vi "pp_loadStimList.vi"(4 "error in (no error)":errorcluster) -> (0 "error out":errorcluster, 2 "Path":path, 3 "Stimulus List":dbl[][](array[numeric]))   [LabVIEW 2013]
uses:
  <vilib>/Utility/xml.llb/Read From XML File(array).vi
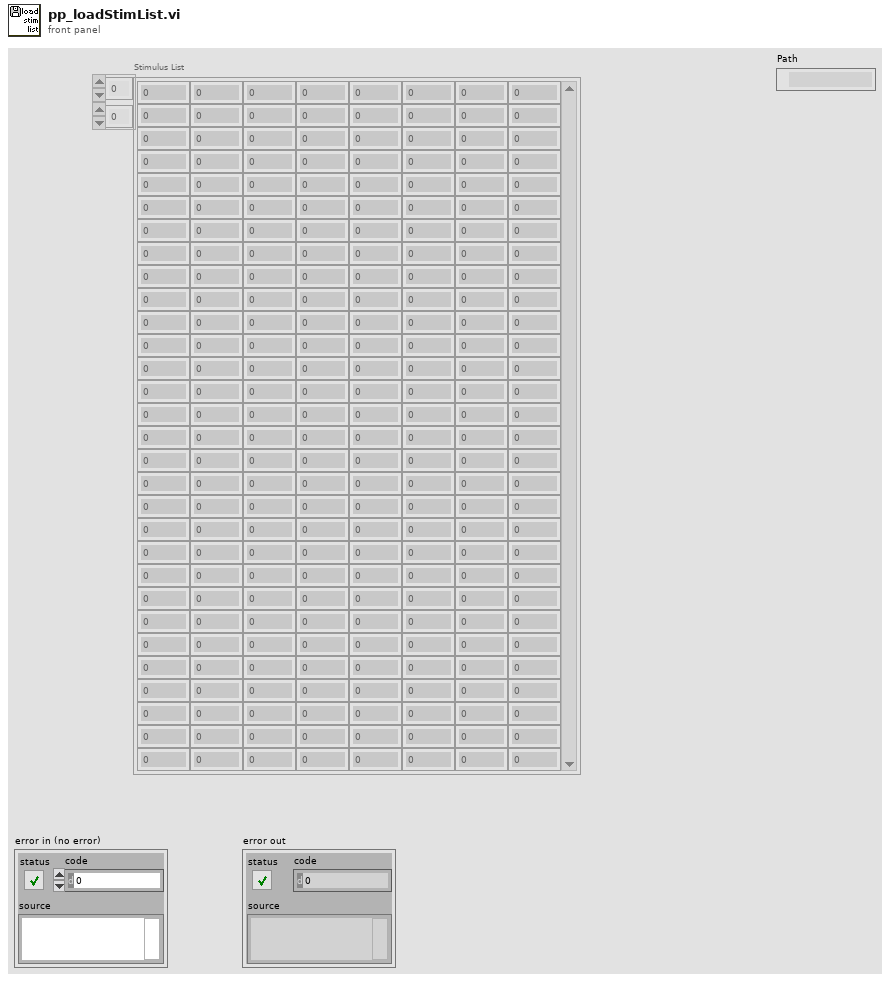
[diagram p1: front panel]
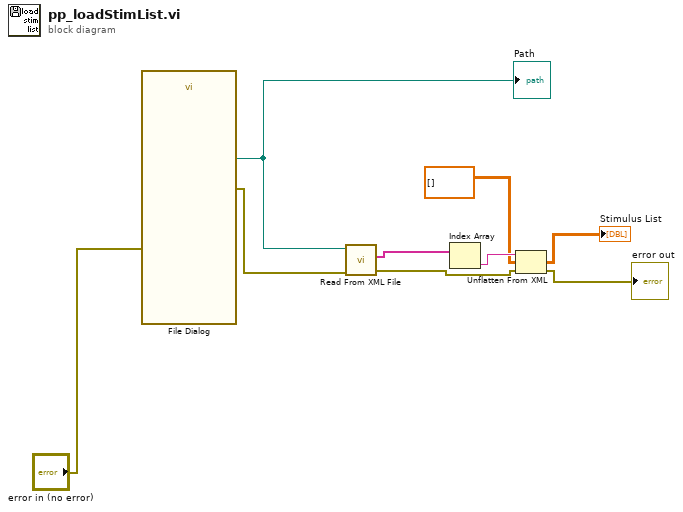
[diagram p0: block diagram]
diagram:
  n1 = call "File Dialog"("error in"="error in (no error)") -> ("selected path"=w8:path, "error out"=w2:errorcluster)  [unwired: 11 in, 2 out]
  "Path" <- w8
  n2 = call-poly <vilib>:"Read From XML File.vi"("error in (no error)"=w2, "XML File Path"=w8) -> ("error out"=w3:errorcluster, "XML Elements"=w7:string[])  [unwired: 7 in, 1 out]
  n3 = Index Array(array=w7) -> (element=w6:string)  [unwired: 1 in]
  n4 = Unflatten From XML(xml string=w6, type=dbl[][] [] ("Stims 1"), error in (no error)=w3) -> (value=→"Stimulus List":dbl[][], error out=→"error out":errorcluster)
